vi "ex 3.2.vi"() -> ()   [LabVIEW 2019]
panel:
  in  "stop":bool
  out "G":bool
  out "F":bool
  out "E":bool
  out "D":bool
  out "C":bool
  out "B":bool
  out "A":bool
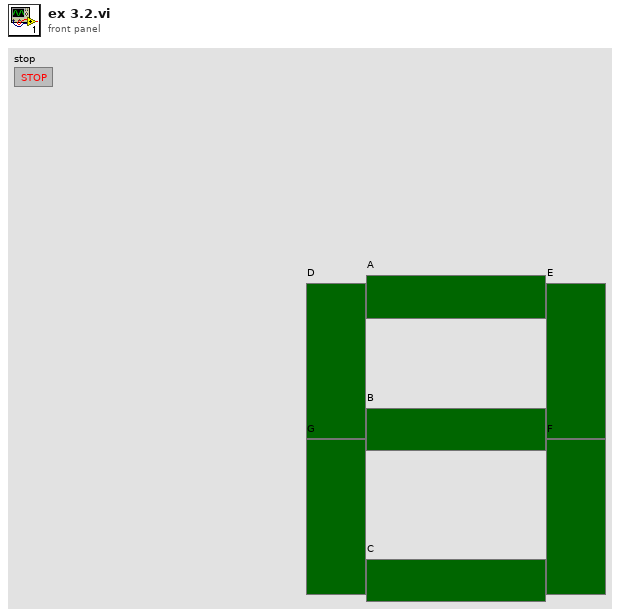
[diagram p1: front panel]
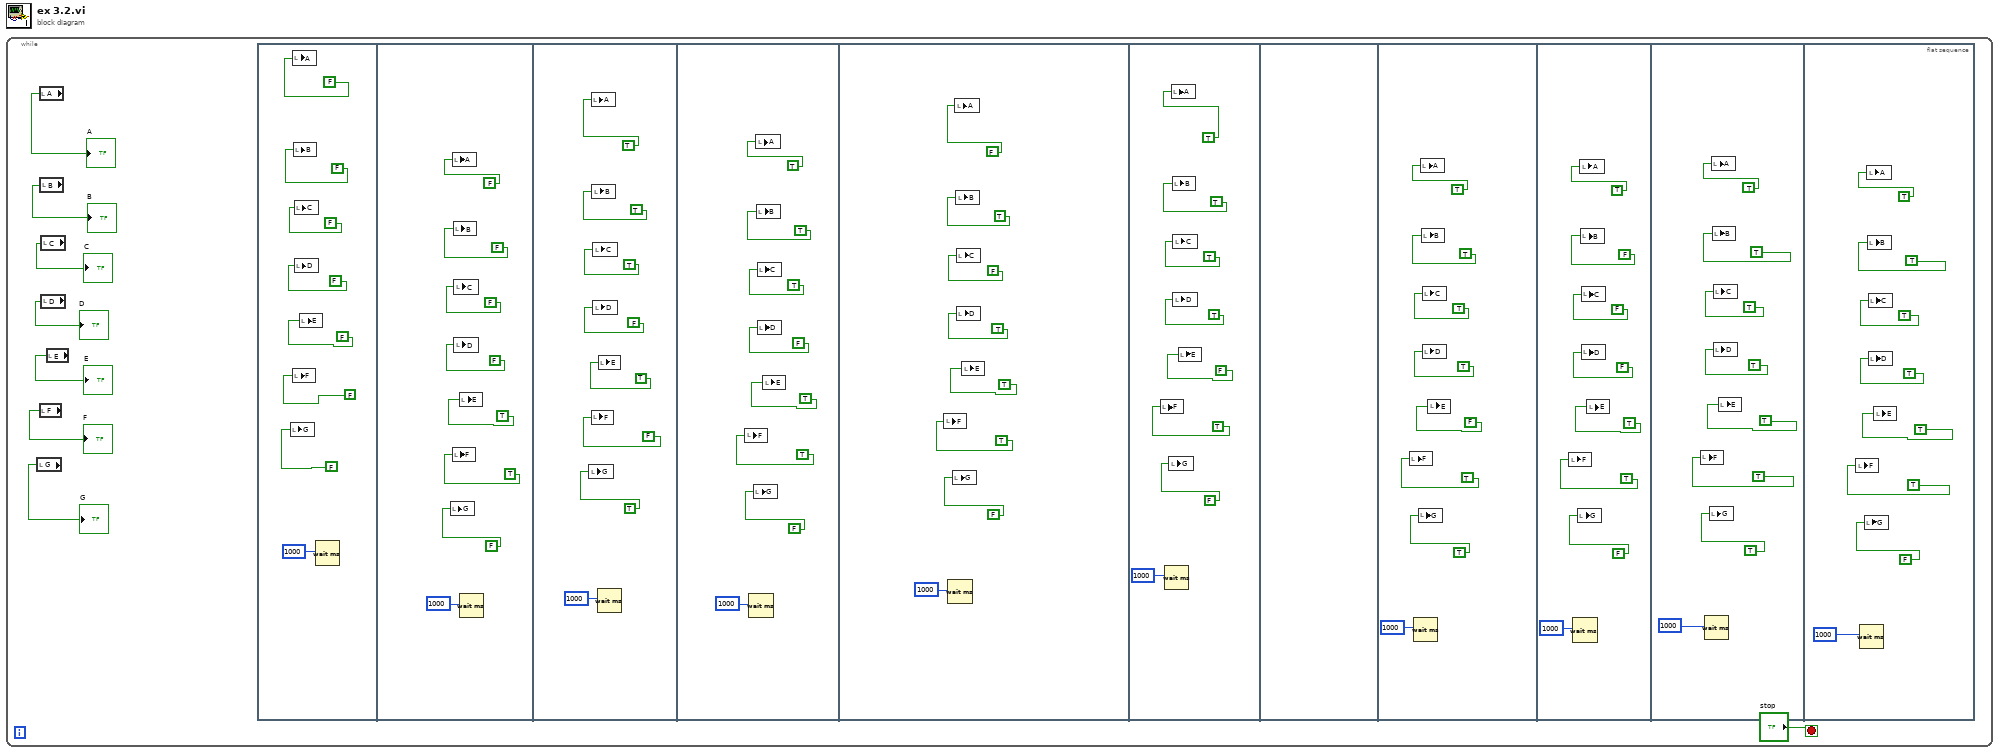
[diagram p0: block diagram]
diagram:
  n1 = while {
    stop <- "stop" stop-if-true
    n2 = local read "G"() -> (→"G":bool)
    n3 = local read "A"() -> (→"A":bool)
    n4 = local read "F"() -> (→"F":bool)
    n5 = local read "B"() -> (→"B":bool)
    n6 = local read "C"() -> (→"C":bool)
    n7 = local read "D"() -> (→"D":bool)
    n8 = local read "E"() -> (→"E":bool)
    n9 = flat-sequence {
      frame #0 {
        n10 = local write "G"(FALSE ("G")) -> ()
        n11 = local write "A"(FALSE ("A")) -> ()
        n12 = local write "F"(FALSE ("F")) -> ()
        n13 = local write "B"(FALSE ("B")) -> ()
        n14 = local write "C"(FALSE ("C")) -> ()
        n15 = local write "D"(FALSE ("D")) -> ()
        n16 = local write "E"(FALSE ("E")) -> ()
        n17 = Wait (ms)(milliseconds to wait=1000) -> ()  [unwired: 1 out]
      }
      frame #1 {
        n18 = local write "G"(FALSE ("G")) -> ()
        n19 = local write "A"(FALSE ("A")) -> ()
        n20 = local write "F"(TRUE ("F")) -> ()
        n21 = local write "B"(FALSE ("B")) -> ()
        n22 = local write "C"(FALSE ("C")) -> ()
        n23 = local write "D"(FALSE ("D")) -> ()
        n24 = local write "E"(TRUE ("E")) -> ()
        n25 = Wait (ms)(milliseconds to wait=1000) -> ()  [unwired: 1 out]
      }
      frame #2 {
        n26 = local write "G"(TRUE ("G")) -> ()
        n27 = local write "A"(TRUE ("A")) -> ()
        n28 = local write "F"(FALSE ("F")) -> ()
        n29 = local write "B"(TRUE ("B")) -> ()
        n30 = local write "C"(TRUE ("C")) -> ()
        n31 = local write "D"(FALSE ("D")) -> ()
        n32 = Wait (ms)(milliseconds to wait=1000) -> ()  [unwired: 1 out]
        n33 = local write "E"(TRUE ("E")) -> ()
      }
      frame #3 {
        n34 = local write "F"(TRUE ("F")) -> ()
        n35 = Wait (ms)(milliseconds to wait=1000) -> ()  [unwired: 1 out]
        n36 = local write "G"(FALSE ("G")) -> ()
        n37 = local write "A"(TRUE ("A")) -> ()
        n38 = local write "B"(TRUE ("B")) -> ()
        n39 = local write "C"(TRUE ("C")) -> ()
        n40 = local write "D"(FALSE ("D")) -> ()
        n41 = local write "E"(TRUE ("E")) -> ()
      }
      frame #4 {
        n42 = local write "F"(TRUE ("F")) -> ()
        n43 = Wait (ms)(milliseconds to wait=1000) -> ()  [unwired: 1 out]
        n44 = local write "G"(FALSE ("G")) -> ()
        n45 = local write "A"(FALSE ("A")) -> ()
        n46 = local write "B"(TRUE ("B")) -> ()
        n47 = local write "C"(FALSE ("C")) -> ()
        n48 = local write "D"(TRUE ("D")) -> ()
        n49 = local write "E"(TRUE ("E")) -> ()
      }
      frame #5 {
        n50 = local write "F"(TRUE ("F")) -> ()
        n51 = Wait (ms)(milliseconds to wait=1000) -> ()  [unwired: 1 out]
        n52 = local write "G"(FALSE ("G")) -> ()
        n53 = local write "A"(TRUE ("A")) -> ()
        n54 = local write "B"(TRUE ("B")) -> ()
        n55 = local write "C"(TRUE ("C")) -> ()
        n56 = local write "D"(TRUE ("D")) -> ()
        n57 = local write "E"(FALSE ("E")) -> ()
      }
      frame #6 {
      }
      frame #7 {
        n58 = local write "F"(TRUE ("F")) -> ()
        n59 = Wait (ms)(milliseconds to wait=1000) -> ()  [unwired: 1 out]
        n60 = local write "G"(TRUE ("G")) -> ()
        n61 = local write "A"(TRUE ("A")) -> ()
        n62 = local write "B"(TRUE ("B")) -> ()
        n63 = local write "C"(TRUE ("C")) -> ()
        n64 = local write "D"(TRUE ("D")) -> ()
        n65 = local write "E"(FALSE ("E")) -> ()
      }
      frame #8 {
        n66 = local write "F"(TRUE ("F")) -> ()
        n67 = Wait (ms)(milliseconds to wait=1000) -> ()  [unwired: 1 out]
        n68 = local write "G"(FALSE ("G")) -> ()
        n69 = local write "A"(TRUE ("A")) -> ()
        n70 = local write "B"(FALSE ("B")) -> ()
        n71 = local write "C"(FALSE ("C")) -> ()
        n72 = local write "D"(FALSE ("D")) -> ()
        n73 = local write "E"(TRUE ("E")) -> ()
      }
      frame #9 {
        n74 = local write "F"(TRUE ("F")) -> ()
        n75 = Wait (ms)(milliseconds to wait=1000) -> ()  [unwired: 1 out]
        n76 = local write "G"(TRUE ("G")) -> ()
        n77 = local write "A"(TRUE ("A")) -> ()
        n78 = local write "B"(TRUE ("B")) -> ()
        n79 = local write "C"(TRUE ("C")) -> ()
        n80 = local write "D"(TRUE ("D")) -> ()
        n81 = local write "E"(TRUE ("E")) -> ()
      }
      frame #10 {
        n82 = local write "F"(TRUE ("F")) -> ()
        n83 = Wait (ms)(milliseconds to wait=1000) -> ()  [unwired: 1 out]
        n84 = local write "G"(FALSE ("G")) -> ()
        n85 = local write "A"(TRUE ("A")) -> ()
        n86 = local write "B"(TRUE ("B")) -> ()
        n87 = local write "C"(TRUE ("C")) -> ()
        n88 = local write "D"(TRUE ("D")) -> ()
        n89 = local write "E"(TRUE ("E")) -> ()
      }
    }
  }
